vi "Generate Pulse Indexies.vi"(4 "dt":dbl, 5 "Size":i32, 6 "t0":timestamp, 7 "Delay":dbl format="%#_6p", 11 "I-V parameters":T1={"Start magnitude"=0.01, "Magnitude increment"=0.001, "End magnitude"=8.0, "Baseline length"=480, "Ramp length"=32, "Top  length"=480, "Threshold "=1e-05, "Processing delay"=25, "Valhalla range"=0.001, "Interpolation"=64} {"Valhalla range" format="%#_6pA"; "Processing delay" format="%dpts"; "Threshold" format="%#_6pV"; "Top  length" format="%dpts"; "Ramp length" format="%dpts"; "Baseline length" format="%dpts"; "End magnitude" format="%#_6pA"; "Magnitude increment" format="%#_6pA"; "Start magnitude" format="%#_6pA"}) -> (3 "Pulse indexies out":T2[](array[typedef]))   [LabVIEW 2016]
uses:
  Pulse indexies.ctl
  I-V parameters.ctl
panel:
  out "32bit integer 2":i32
  out "Single pulse length":i32
  out "32bit integer":T3
  in  "Pulse indexies":T2
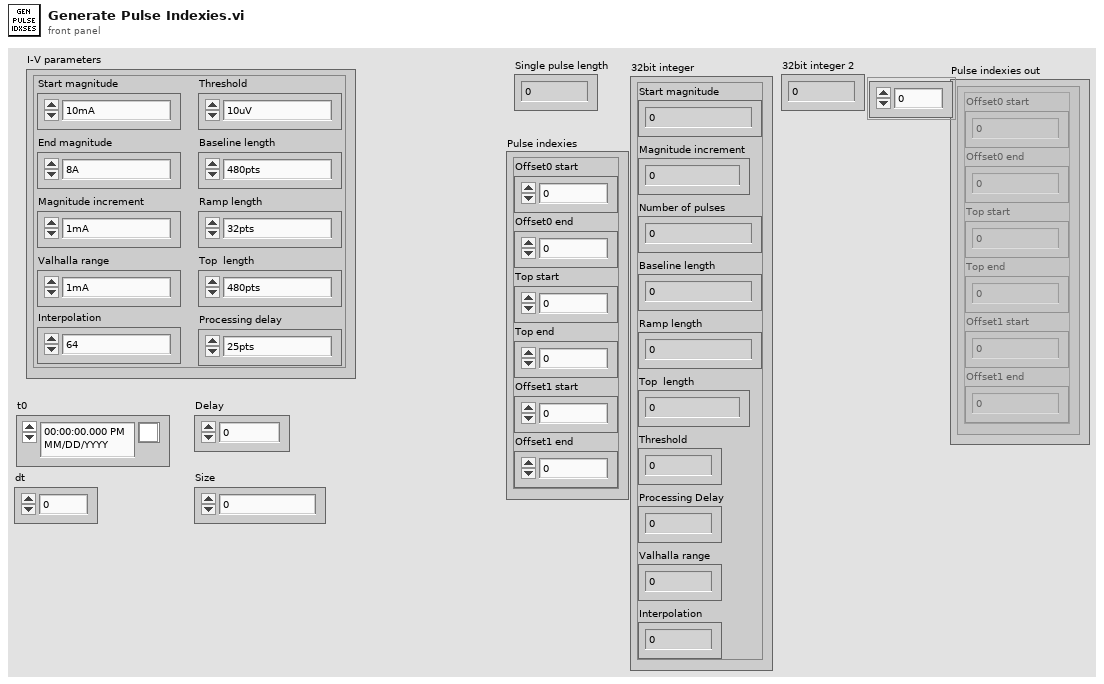
[diagram p1: front panel]
types:
  T1 = typedef "I-V parameters.ctl" = cluster{"Start magnitude":dbl, "Magnitude increment":dbl, "End magnitude":dbl, "Baseline length":i32, "Ramp length":i32, "Top  length":i32, "Threshold ":dbl, "Processing delay":u16, "Valhalla range":dbl, "Interpolation":i32}
  T2 = typedef "Pulse indexies.ctl" = cluster{"Offset0 start ":i32, "Offset0 end":i32, "Top start":i32, "Top end":i32, "Offset1 start":i32, "Offset1 end":i32}
  T3 = cluster{"Start magnitude":i32, "Magnitude increment":i32, "Number of pulses":i32, "Baseline length":i32, "Ramp length":i32, "Top  length":i32, "Threshold ":i32, "Processing Delay":i32, "Valhalla range":i32, "Interpolation":i32}
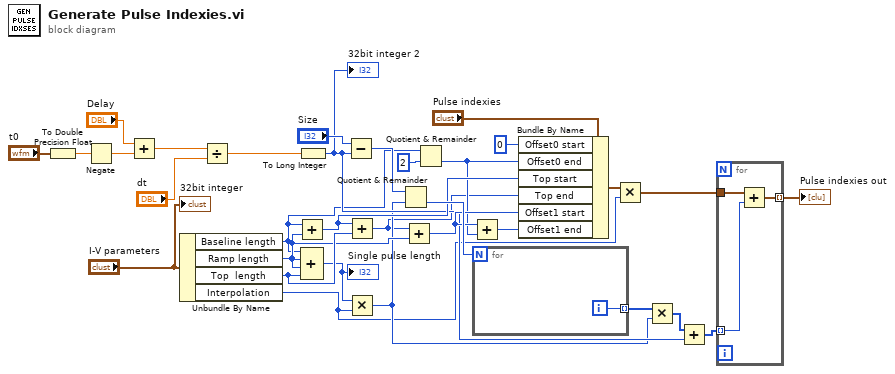
[diagram p0: block diagram]
diagram:
  n1 = To Double Precision Float(number="t0") -> (double precision float=w31:dbl)
  n2 = Negate(x=w31) -> (-x=w30:dbl)
  n3 = Add(x="Delay", y=w30) -> (x+y=w28:dbl)
  n4 = Unbundle By Name("I-V parameters") -> ("Baseline length"=w6:i32, "Ramp length"=w18:i32, "Top  length"=w19:i32, "Interpolation"=w2:i32)
  n5 = Divide(x=w28, y="dt") -> (x/y=w27:dbl)
  n6 = Add(x=w6, y=w18) -> (x+y=w20:i32)
  n7 = To Long Integer(number=w27) -> (32bit integer=w14:i32)
  "32bit integer 2" <- w14
  n8 = Compound Arithmetic op=ADD(w6, w18, w18, w19) -> (w3:i32)
  "Single pulse length" <- w3
  n9 = Subtract(x="Size", y=w14) -> (x-y=w25:i32)
  n10 = Add(x=w20, y=w19) -> (x+y=w1:i32)
  n11 = Multiply(x=w3, y=w2) -> (x*y=w7:i32)
  n12 = Quotient & Remainder(x=w25, y=w7) -> (floor(x/y)=w24:i32)  [unwired: 1 out]
  n13 = Add(x=w1, y=w18) -> (x+y=w17:i32)
  n14 = Quotient & Remainder(x=w6, y=2) -> (floor(x/y)=w5:i32)  [unwired: 1 out]
  n15 = Add(x=w17, y=w5) -> (x+y=w16:i32)
  n16 = for {
    N: w24 -> [_]
    tunnel: [w33] -> w15 mode=indexing
    i -> [w33]
  }
  n17 = Bundle By Name(cluster="Pulse indexies", "Offset0 start"=0, "Offset0 end"=w5, "Top start"=w20, "Top end"=w1, "Offset1 start"=w17, "Offset1 end"=w16) -> (w8:T2)
  n18 = Multiply(x=w8, y=w2) -> (x*y=w9:T2)
  n19 = Multiply(x=w15, y=w7) -> (x*y=w13:i32[])
  n20 = Add(x=w13, y=w14) -> (x+y=w12:i32[])
  n21 = for {
    tunnel: w12 -> [w36] mode=indexing
    tunnel: w9 -> [w35]
    tunnel: [w34] -> w11 mode=indexing
    n22 = Add(x=w35, y=w36) -> (x+y=w34:T2)
  }
  "Pulse indexies out" <- w11
  "32bit integer" <- "I-V parameters"
